vi "Draw RangeArrows.vi"(4 "Vertical":bool, 6 "pen":T1, 9 "Color":u32, 10 "position":T2, 11 "picture":picture) -> (3 "new picture":picture)   [LabVIEW 2020, in "GarphView.lvlib" / "GarphView.lvclass"]
doc: "Draw the crossing lines for ranges, either vertically or horizontally."
uses:
  GarphView.lvclass
  <vilib>/Utility/miscctls.llb/LVPoint32TypeDef.ctl
  GarphView.lvclass/GarphView.ctl
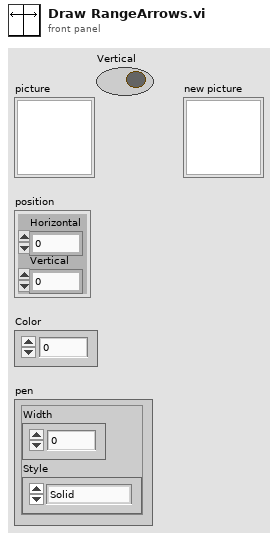
[diagram p1: front panel]
types:
  T1 = cluster{"Width":u16, "Style":enum32{"Solid", "Dash", "Dot", "DashDot", "DashDotDot"}}
  T2 = typedef "LVPoint32TypeDef.ctl" = cluster{"Horizontal":i32, "Vertical":i32}
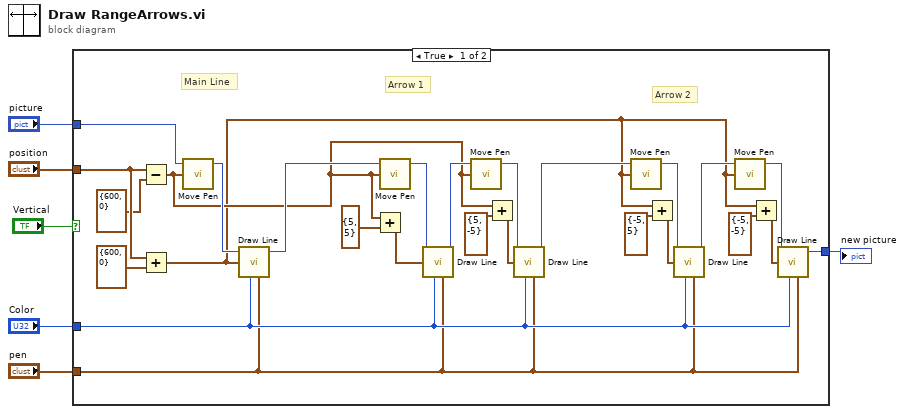
[diagram p0: block diagram]
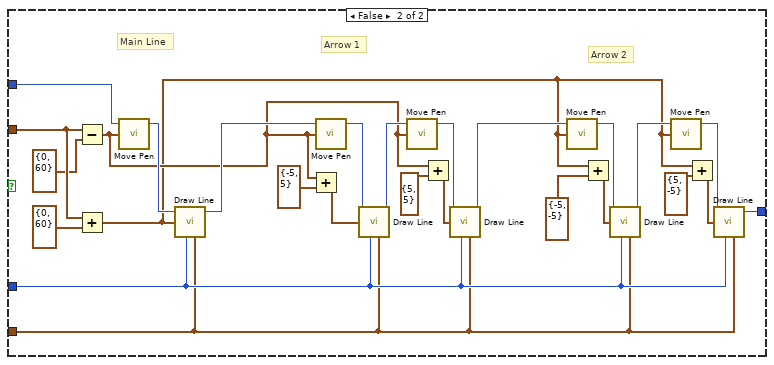
[diagram p2: hidden frame]
diagram:
  n1 = case shown="True" "Vertical" {
    tunnel: "position" -> [w31 w57]
    tunnel: "picture" -> [w29 w55]
    tunnel: "Color" -> [w9 w35]
    tunnel: "pen" -> [w8 w34]
    tunnel: [w7 w33] -> w2
    frame True {
      # "Arrow 2"
      # "Arrow 1"
      # "Main Line"
      n2 = Subtract(x=w31, y=T2 {"Horizontal"=600, "Vertical"=0}) -> (x-y=w21:T2)
      n3 = Add(x=w31, y=T2 {"Horizontal"=600, "Vertical"=0}) -> (x+y=w10:T2)
      n4 = call <vilib>:"Move Pen.vi"("new position"=w21, "picture"=w29) -> ("new picture"=w28:picture)  [unwired: 3 in]
      n5 = call <vilib>:"Draw Line.vi"("picture"=w28, "end point"=w10, "color(black)"=w9, "pen"=w8) -> ("new picture"=w27:picture)  [unwired: 5 in]
      n6 = Add(x=w21, y=T2 {"Horizontal"=5, "Vertical"=5}) -> (x+y=w25:T2)
      n7 = call <vilib>:"Move Pen.vi"("new position"=w21, "picture"=w27) -> ("new picture"=w24:picture)  [unwired: 3 in]
      n8 = call <vilib>:"Draw Line.vi"("picture"=w24, "end point"=w25, "color(black)"=w9, "pen"=w8) -> ("new picture"=w23:picture)  [unwired: 5 in]
      n9 = call <vilib>:"Move Pen.vi"("new position"=w21, "picture"=w23) -> ("new picture"=w22:picture)  [unwired: 3 in]
      n10 = Add(x=w21, y=T2 {"Horizontal"=5, "Vertical"=-5}) -> (x+y=w19:T2)
      n11 = call <vilib>:"Draw Line.vi"("picture"=w22, "end point"=w19, "color(black)"=w9, "pen"=w8) -> ("new picture"=w15:picture)  [unwired: 5 in]
      n12 = call <vilib>:"Move Pen.vi"("new position"=w10, "picture"=w15) -> ("new picture"=w16:picture)  [unwired: 3 in]
      n13 = Add(x=w10, y=T2 {"Horizontal"=-5, "Vertical"=5}) -> (x+y=w18:T2)
      n14 = call <vilib>:"Draw Line.vi"("picture"=w16, "end point"=w18, "color(black)"=w9, "pen"=w8) -> ("new picture"=w11:picture)  [unwired: 5 in]
      n15 = call <vilib>:"Move Pen.vi"("new position"=w10, "picture"=w11) -> ("new picture"=w14:picture)  [unwired: 3 in]
      n16 = Add(x=w10, y=T2 {"Horizontal"=-5, "Vertical"=-5}) -> (x+y=w12:T2)
      n17 = call <vilib>:"Draw Line.vi"("picture"=w14, "end point"=w12, "color(black)"=w9, "pen"=w8) -> ("new picture"=w7:picture)  [unwired: 5 in]
    }
    frame False {
      # "Arrow 2"
      # "Arrow 1"
      # "Main Line"
      n18 = Subtract(x=w57, y=T2 {"Horizontal"=0, "Vertical"=60}) -> (x-y=w47:T2)
      n19 = Add(x=w57, y=T2 {"Horizontal"=0, "Vertical"=60}) -> (x+y=w36:T2)
      n20 = call <vilib>:"Move Pen.vi"("new position"=w47, "picture"=w55) -> ("new picture"=w54:picture)  [unwired: 3 in]
      n21 = call <vilib>:"Draw Line.vi"("picture"=w54, "end point"=w36, "color(black)"=w35, "pen"=w34) -> ("new picture"=w53:picture)  [unwired: 5 in]
      n22 = Add(x=w47, y=T2 {"Horizontal"=-5, "Vertical"=5}) -> (x+y=w51:T2)
      n23 = call <vilib>:"Move Pen.vi"("new position"=w47, "picture"=w53) -> ("new picture"=w50:picture)  [unwired: 3 in]
      n24 = call <vilib>:"Draw Line.vi"("picture"=w50, "end point"=w51, "color(black)"=w35, "pen"=w34) -> ("new picture"=w49:picture)  [unwired: 5 in]
      n25 = call <vilib>:"Move Pen.vi"("new position"=w47, "picture"=w49) -> ("new picture"=w48:picture)  [unwired: 3 in]
      n26 = Add(x=w47, y=T2 {"Horizontal"=5, "Vertical"=5}) -> (x+y=w45:T2)
      n27 = call <vilib>:"Draw Line.vi"("picture"=w48, "end point"=w45, "color(black)"=w35, "pen"=w34) -> ("new picture"=w41:picture)  [unwired: 5 in]
      n28 = call <vilib>:"Move Pen.vi"("new position"=w36, "picture"=w41) -> ("new picture"=w42:picture)  [unwired: 3 in]
      n29 = Add(x=w36, y=T2 {"Horizontal"=-5, "Vertical"=-5}) -> (x+y=w44:T2)
      n30 = call <vilib>:"Draw Line.vi"("picture"=w42, "end point"=w44, "color(black)"=w35, "pen"=w34) -> ("new picture"=w37:picture)  [unwired: 5 in]
      n31 = call <vilib>:"Move Pen.vi"("new position"=w36, "picture"=w37) -> ("new picture"=w40:picture)  [unwired: 3 in]
      n32 = Add(x=w36, y=T2 {"Horizontal"=5, "Vertical"=-5}) -> (x+y=w38:T2)
      n33 = call <vilib>:"Draw Line.vi"("picture"=w40, "end point"=w38, "color(black)"=w35, "pen"=w34) -> ("new picture"=w33:picture)  [unwired: 5 in]
    }
  }
  "new picture" <- w2
